vi "Periodic Tasks.vi"(8 "error in":errorcluster) -> ()   [LabVIEW 2017]
doc: "This VI runs in parallel to other tasks. It can contain as many user-defined periodic loops as you need. These can carry out PID or other sorts of timed response."
uses:
  <vilib>/Rock Robotics/WPI/Solenoid/WPI_SolenoidValue.ctl
  <vilib>/Rock Robotics/WPI/ThirdParty/Phoenix-LabVIEW/Motor Controller/Controls/CTRE_Phoenix_MotorControl_ControlMode.ctl
  <vilib>/Rock Robotics/WPI/ThirdParty/Phoenix-LabVIEW/Pigeon IMU/CTRE_PigeonIMU_TareType.ctl
  <vilib>/Rock Robotics/WPI/Utilities/WPI_GetSetVariantRefNum.vi
  Robot Global Data.vi
  <vilib>/Rock Robotics/Network Tables/NT Read Number.vi
  <vilib>/Rock Robotics/Network Tables/NT Write Number.vi
  <vilib>/Rock Robotics/WPI/ThirdParty/Phoenix-LabVIEW/Pigeon IMU/CTRE_PigeonIMU_GetYPR.vi
  <vilib>/Rock Robotics/WPI/ThirdParty/Phoenix-LabVIEW/Motor Controller/Get/CTRE_Phoenix_MotorController_GetSelectedSensorData.vi
  <vilib>/Rock Robotics/WPI/ThirdParty/Phoenix-LabVIEW/Motor Controller/Get/CTRE_Phoenix_MotorController_GetLimitSwitchStates.vi
  <vilib>/Rock Robotics/WPI/Solenoid/WPI_SolenoidSetEnum.vi
  <vilib>/Utility/file.llb/Read Delimited Spreadsheet (DBL).vi
panel:
  out "all rows":dbl[][](array[numeric])
  out "Waveform Chart":dbl(graph)
  in  "HFB_Duration":dbl=200.0
  out "HFB_Start":dbl
  in  "Throttle Correction":bool=TRUE
  in  "Aim-Assist Gain":dbl=0.6
  out "4":dbl(graph)
  out "Current":dbl(graph)
  out "in":i32
  out "ARM":dbl
  out "FWD":bool
  out "Right spd":dbl
  out "Left spd":dbl
  out "Right pos":i32
  out "Left pos":i32
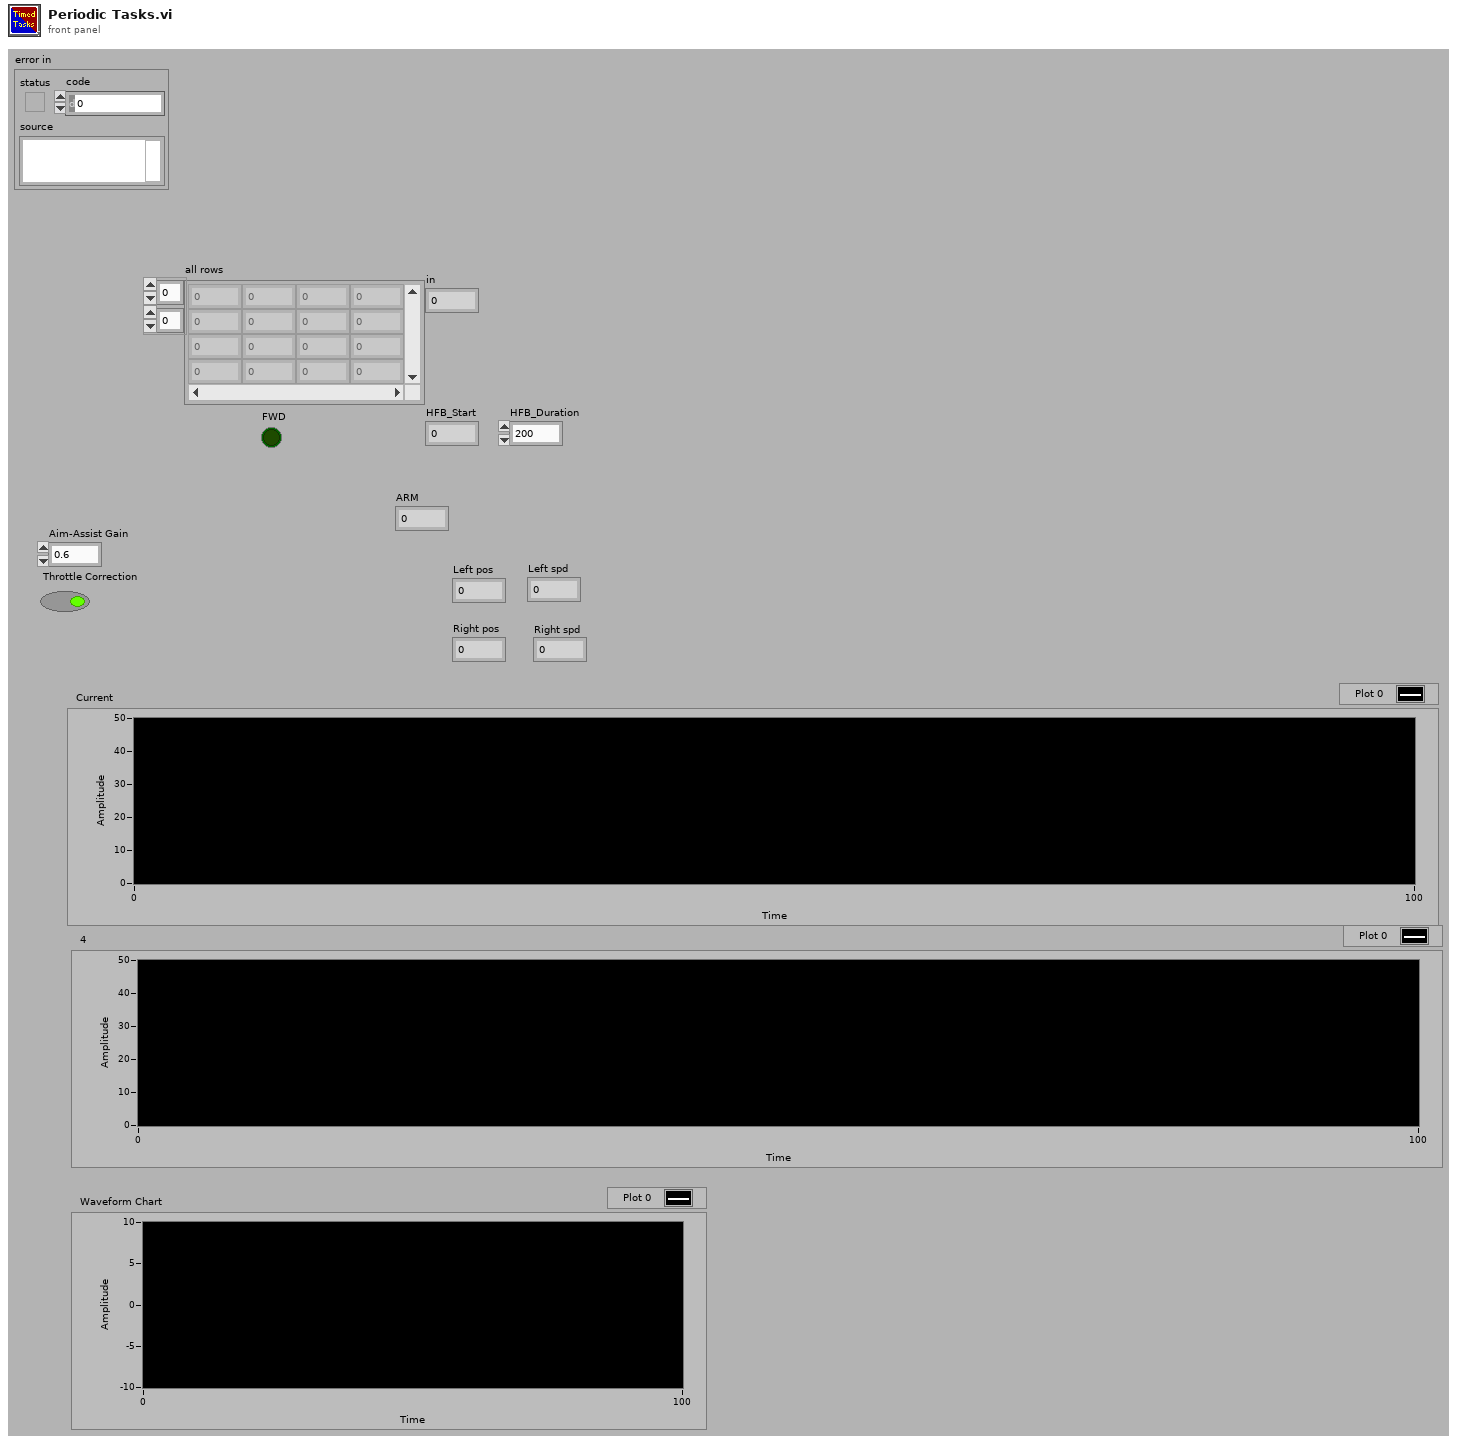
[diagram p1: front panel]
types:
  T1 = typedef "WPI_JoystickDevRef.ctl" = cluster{"Device":T2}
  T2 = typedef "WPI_JoystickDeviceEnum.ctl" = enum16{"USB 0", "USB 1", "USB 2", "USB 3", "USB 4", "USB 5"}
  T3 = typedef "WPI_RobotDriveDevRef.ctl" = cluster{"DevStatus":errorcluster, "Motors[]":T4[], "Square Inputs":bool, "Max Output":dbl}
  T4 = typedef "WPI_MotorControlDeviceRef.ctl" = cluster{"DeviceStatus":errorcluster, "Type":T5, "PWM":cluster{"PWM Channel":T6, "DeadBand":T7}, "CAN":cluster{"Device Number":u8, "SetOutput VI Ref":variant, "GetOutput VI Ref":variant, "Enable VI Ref":variant, "Disable VI Ref":variant, "Data":variant}, "Invert":bool, "DIO PWM":cluster{"PWM \"Enable\" Channel":T6, "DIOChannel":T8, "PWM Rate":dbl}}
  T5 = typedef "WPI_MotorControlType.ctl" = enum16{"PWM", "CAN", "DIO PWM"}
  T6 = typedef "FPGA_DIOPWMChannel.ctl" = enum8{"PWM 0", "PWM 1", "PWM 2", "PWM 3", "PWM 4", "PWM 5", "PWM 6", "PWM 7", "PWM 8", "PWM 9", "PWM MXP 0", "PWM MXP 1", "PWM MXP 2", "PWM MXP 3", "PWM MXP 4", "PWM MXP 5", "PWM MXP 6", "PWM MXP 7", "PWM MXP 8", "PWM MXP 9", "Invalid"}
  T7 = typedef "WPI_PWMDeadband.ctl" = cluster{"Name":string, "maxPositivePwm":i32, "minPositivePwm":i32, "centerPwm":i32, "maxNegativePwm":i32, "minNegativePwm":i32, "angularRange":u16}
  T8 = typedef "FPGA_DIOChannel.ctl" = enum8{"DIO 0", "DIO 1", "DIO 2", "DIO 3", "DIO 4", "DIO 5", "DIO 6", "DIO 7", "DIO 8", "DIO 9", "DIO MXP 0", "DIO MXP 1", "DIO MXP 2", "DIO MXP 3", "DIO MXP 4", "DIO MXP 5", "DIO MXP 6", "DIO MXP 7", "DIO MXP 8", "DIO MXP 9", "DIO MXP 10", "DIO MXP 11", "DIO MXP 12", "DIO MXP 13", "DIO MXP 14", "DIO MXP 15", "SPI Port CS1", "SPI Port CS2", "SPI Port CS3", "SPI Port MISO", "SPI Port MOSI", "Invalid"}
  T9 = typedef "WPI_SolenoidDevRef.ctl" = cluster{"DevStatus":errorcluster, "Pneumatics Control Module":u8, "Forward Solenoid Channel":T10, "Reverse Solenoid Channel":T10}
  T10 = typedef "WPI_SolenoidChannel.ctl" = enum8{"Solenoid 0", "Solenoid 1", "Solenoid 2", "Solenoid 3", "Solenoid 4", "Solenoid 5", "Solenoid 6", "Solenoid 7", "Invalid"}
  T11 = typedef "CTRE_PigeonIMU_DeviceRef.ctl" = cluster{"DeviceStatus":errorcluster, "Device Number":u8, "Type":T12, "Device ID":u32, "Handle":u64, "UsageFrame":u32, "Library Path":path}
  T12 = typedef "CTRE_PigeonIMU_ConnectionType.ctl" = u32
  T13 = cluster{"JoystickDevRef":T1, "JoystickDevRef":T1, "RobotDriveDevRef":T3, "PhoenixMotorControlDevRef":T4, "SolenoidDevRef":T9, "PhoenixMotorControlDevRef":T4, "SolenoidDevRef":T9, "SolenoidDevRef":T9, "PhoenixMotorControlDevRef":T4, "PhoenixMotorControlDevRef":T4, "SolenoidDevRef":T9, "PhoenixMotorControlDevRef":T4, "PhoenixMotorControlDevRef":T4, "PigeonIMUDevRef":T11, "SolenoidDevRef":T9, "Name":string, "Name":string, "Name":string, "Name":string}
  T14 = typedef "CTRE_PigeonIMU_TareType.ctl" = u8
  T15 = typedef "WPI_DriverStationRobotMode2.ctl" = enum16{"Autonomous Disabled", "Autonomous Enabled", "Teleop Disabled", "Teleop Enabled", "Disconnected", "Finish", "Test Disabled", "Test Enabled", "Emergency Stopped"}
  T16 = typedef "WPI_SolenoidValue.ctl" = enum16{"Off", "On", "Forward", "Reverse"}
  T17 = typedef "CTRE_Phoenix_MotorControl_ControlMode.ctl" = u16
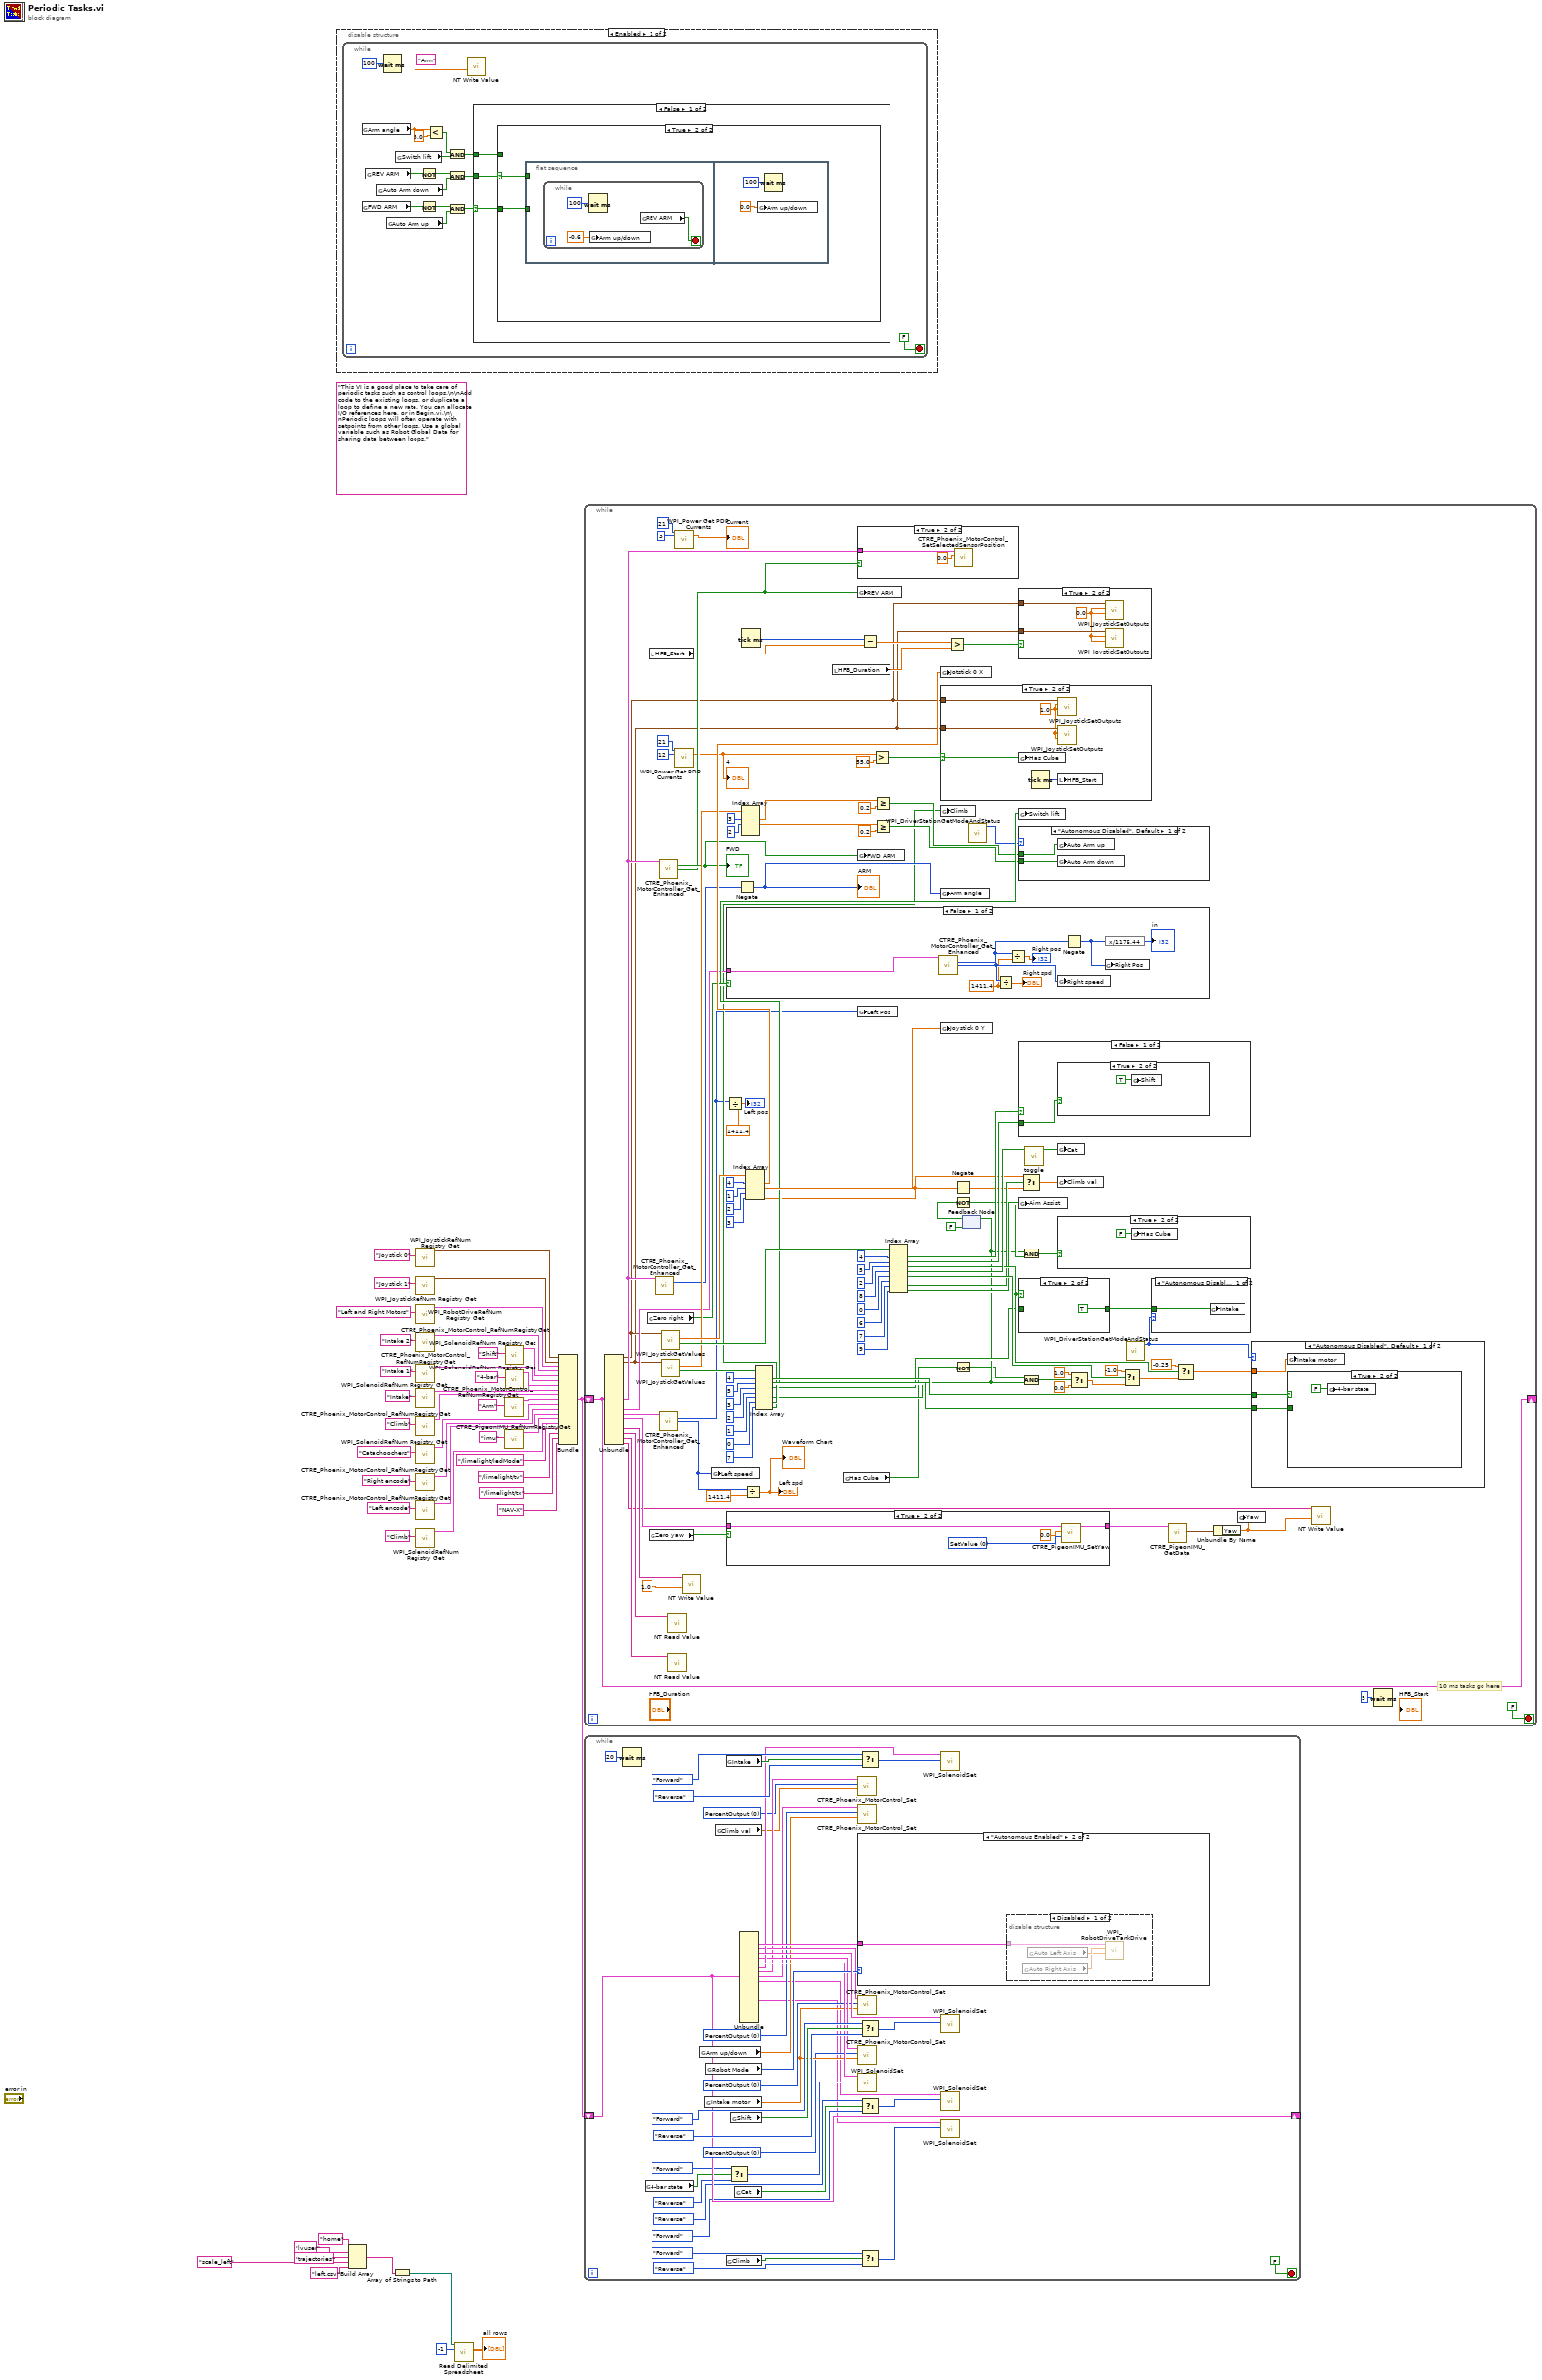
[diagram p0: block diagram]
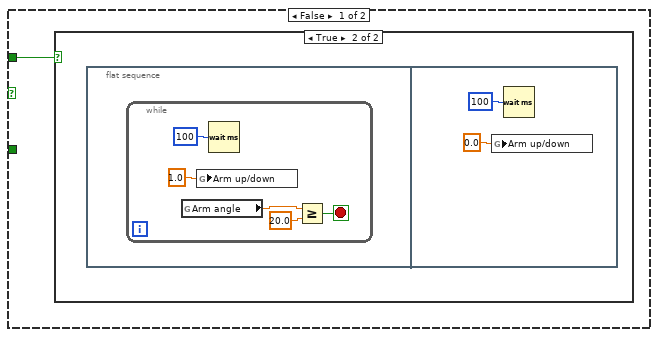
[diagram p2: hidden frame]
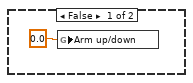
[diagram p3: hidden frame]
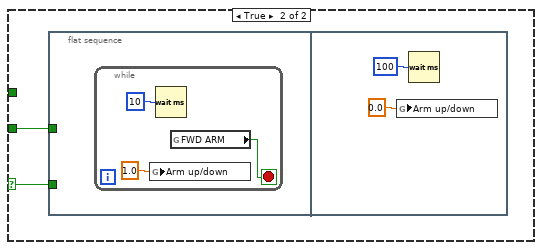
[diagram p4: hidden frame]
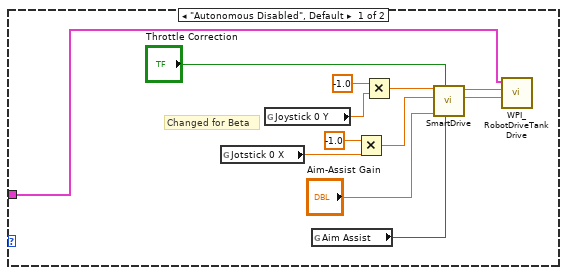
[diagram p6: hidden frame]
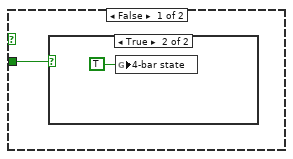
[diagram p14: hidden frame]
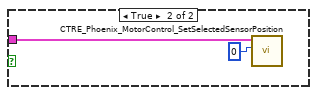
[diagram p19: hidden frame]
diagram:
  (unwired) "This VI is a good place to take care of periodic tasks such as control loops.\n\nAdd code to the existing loops, or duplicate a loop to define a new rate. You can allocate I/O references here, or in Begin.vi.\n\nPeriodic loops will often operate with setpoints from other loops. Use a global variable such as Robot Global Data for sharing data between loops."
  n1 = disable-structure shown="Enabled" {
    frame Enabled {
      n2 = while {
        stop <- FALSE stop-if-true
        n3 = global read "Robot Global Data.vi" "Arm angle"() -> (w54:dbl)
        n4 = global read "Robot Global Data.vi" "FWD ARM"() -> (w46:bool)
        n5 = global read "Robot Global Data.vi" "REV ARM"() -> (w48:bool)
        n6 = global read "Robot Global Data.vi" "Auto Arm down"() -> (w50:bool)
        n7 = Wait (ms)(milliseconds to wait=u32 100) -> ()  [unwired: 1 out]
        n8 = global read "Robot Global Data.vi" "Auto Arm up"() -> (w52:bool)
        n9 = global read "Robot Global Data.vi" "Switch lift"() -> (w56:bool)
        n10 = Not(x=w48) -> (.not. x?=w47:bool)
        n11 = Not(x=w46) -> (.not. x?=w45:bool)
        n12 = Less?(x=w54, y=5.0) -> (x < y?=w57:bool)
        n13 = And(x=w57, y=w56) -> (x .and. y?=w55:bool)
        n14 = Compound Arithmetic op=AND(w47, w50) -> (w49:bool)
        n15 = Compound Arithmetic op=AND(w45, w52) -> (w51:bool)
        n16 = call-poly <vilib>:"NT Write Value.vi"("Numeric"=w54, "Name"="Arm") -> ()  [unwired: 9 in, 1 out]
        n17 = case shown="False" w51 {
          selector: w51 -> [w62 w80]
          tunnel: w49 -> [w63 w81]
          tunnel: w55 -> [w61 _]
          frame False {
            n18 = case shown="True" w63 {
              selector: w63 -> [_ w74]
              tunnel: w62 -> [_ w73]
              tunnel: w61 -> [w64 _]
              frame False {
                n19 = case shown="True" w64 {
                  frame False {
                    n20 = global write "Robot Global Data.vi" "Arm up/down"(0.0 ("Arm up/down")) -> ()
                  }
                  frame True {
                    n21 = flat-sequence {
                      frame #0 {
                        n22 = while {
                          stop <- w67 stop-if-true
                          n23 = global read "Robot Global Data.vi" "Arm angle"() -> (w69:dbl)
                          n24 = global write "Robot Global Data.vi" "Arm up/down"(1.0) -> ()
                          n25 = Wait (ms)(milliseconds to wait=u32 100) -> ()  [unwired: 1 out]
                          n26 = Greater Or Equal?(x=w69, y=20.0) -> (x >= y?=w67:bool)
                        }
                      }
                      frame #1 {
                        n27 = global write "Robot Global Data.vi" "Arm up/down"(0.0) -> ()
                        n28 = Wait (ms)(milliseconds to wait=u32 100) -> ()  [unwired: 1 out]
                      }
                    }
                  }
                }
              }
              frame True {
                n29 = flat-sequence {
                  tunnel: w74 -> [_]
                  tunnel: w73 -> [_]
                  frame #0 {
                    n30 = while {
                      stop <- w75 stop-if-true
                      n31 = Wait (ms)(milliseconds to wait=u32 100) -> ()  [unwired: 1 out]
                      n32 = global write "Robot Global Data.vi" "Arm up/down"(-0.6) -> ()
                      n33 = global read "Robot Global Data.vi" "REV ARM"() -> (w75:bool)
                    }
                  }
                  frame #1 {
                    n34 = global write "Robot Global Data.vi" "Arm up/down"(0.0) -> ()
                    n35 = Wait (ms)(milliseconds to wait=u32 100) -> ()  [unwired: 1 out]
                  }
                }
              }
            }
          }
          frame True {
            n36 = flat-sequence {
              tunnel: w81 -> [_]
              tunnel: w80 -> [_]
              frame #0 {
                n37 = while {
                  stop <- w82 stop-if-true
                  n38 = global write "Robot Global Data.vi" "Arm up/down"(1.0) -> ()
                  n39 = Wait (ms)(milliseconds to wait=u32 10) -> ()  [unwired: 1 out]
                  n40 = global read "Robot Global Data.vi" "FWD ARM"() -> (w82:bool)
                }
              }
              frame #1 {
                n41 = global write "Robot Global Data.vi" "Arm up/down"(0.0) -> ()
                n42 = Wait (ms)(milliseconds to wait=u32 100) -> ()  [unwired: 1 out]
              }
            }
          }
        }
      }
    }
    frame Disabled {
    }
  }
  n43 = Build Array("home", "lvuser" ("element"), "trajectories" ("element"), "scale_left" ("element"), "left.csv" ("element")) -> (w3:string[])
  n44 = Array of Strings to Path(0:w3) -> (2:w2:path)  [unwired: 1 in]
  n45 = call <vilib>:"WPI_JoystickRefNum Registry Get.vi"("refnum name"="Joystick 0") -> ("JoystickDevRef"=w32:T1)  [unwired: 1 in, 9 out]
  n46 = call <vilib>:"WPI_JoystickRefNum Registry Get.vi"("refnum name"="Joystick 1") -> ("JoystickDevRef"=w42:T1)  [unwired: 1 in, 9 out]
  n47 = call <vilib>:"WPI_RobotDriveRefNum Registry Get.vi"("refnum name"="Left and Right Motors") -> ("RobotDriveDevRef"=w41:T3)  [unwired: 1 in, 9 out]
  n48 = call <vilib>:"CTRE_Phoenix_MotorControl_RefNumRegistryGet.vi"("refnum name"="Intake 2") -> ("PhoenixMotorControlDevRef"=w38:T4)  [unwired: 9 in, 1 out]
  n49 = call <vilib>:"CTRE_Phoenix_MotorControl_RefNumRegistryGet.vi"("refnum name"="Intake 1") -> ("PhoenixMotorControlDevRef"=w35:T4)  [unwired: 9 in, 1 out]
  n50 = call <vilib>:"WPI_SolenoidRefNum Registry Get.vi"("refnum name"="Intake") -> ("SolenoidDevRef"=w30:T9)  [unwired: 9 in, 1 out]
  n51 = call <vilib>:"CTRE_Phoenix_MotorControl_RefNumRegistryGet.vi"("refnum name"="Climb") -> ("PhoenixMotorControlDevRef"=w26:T4)  [unwired: 9 in, 1 out]
  n52 = call <vilib>:"WPI_SolenoidRefNum Registry Get.vi"("refnum name"="Catachoochers") -> ("SolenoidDevRef"=w22:T9)  [unwired: 9 in, 1 out]
  n53 = call <vilib>:"CTRE_Phoenix_MotorControl_RefNumRegistryGet.vi"("refnum name"="Right encode") -> ("PhoenixMotorControlDevRef"=w20:T4)  [unwired: 9 in, 1 out]
  n54 = call <vilib>:"CTRE_Phoenix_MotorControl_RefNumRegistryGet.vi"("refnum name"="Left encode") -> ("PhoenixMotorControlDevRef"=w18:T4)  [unwired: 9 in, 1 out]
  n55 = call <vilib>:"WPI_SolenoidRefNum Registry Get.vi"("refnum name"="Climb") -> ("SolenoidDevRef"=w14:T9)  [unwired: 9 in, 1 out]
  n56 = call-poly <vilib>:"Read Delimited Spreadsheet.vi"("file path (dialog if empty)"=w2, "number of rows (all:-1)"=-1) -> ("all rows"=→"all rows":dbl[][])  [unwired: 8 in, 5 out]
  n57 = call <vilib>:"CTRE_Phoenix_MotorControl_RefNumRegistryGet.vi"("refnum name"="Arm") -> ("PhoenixMotorControlDevRef"=w24:T4)  [unwired: 9 in, 1 out]
  n58 = call <vilib>:"CTRE_PigeonIMU_RefNumRegistryGet.vi"("refnum name"="imu") -> ("PigeonIMUDevRef"=w17:T11)  [unwired: 9 in, 1 out]
  n59 = call <vilib>:"WPI_SolenoidRefNum Registry Get.vi"("refnum name"="Shift") -> ("SolenoidDevRef"=w36:T9)  [unwired: 9 in, 1 out]
  n60 = call <vilib>:"WPI_SolenoidRefNum Registry Get.vi"("refnum name"="4-bar") -> ("SolenoidDevRef"=w31:T9)  [unwired: 9 in, 1 out]
  n61 = Bundle("JoystickDevRef"=w32, "JoystickDevRef"=w42, "RobotDriveDevRef"=w41, "PhoenixMotorControlDevRef"=w38, "SolenoidDevRef"=w36, "PhoenixMotorControlDevRef"=w35, "SolenoidDevRef"=w31, "SolenoidDevRef"=w30, "PhoenixMotorControlDevRef"=w26, "PhoenixMotorControlDevRef"=w24, "SolenoidDevRef"=w22, "PhoenixMotorControlDevRef"=w20, "PhoenixMotorControlDevRef"=w18, "PigeonIMUDevRef"=w17, "SolenoidDevRef"=w14, "Name"="/limelight/ledMode", "Name"="/limelight/tv", "Name"="/limelight/tx", "Name"="NAV-X") -> (w40:T13)  [unwired: 1 out]
  n62 = while {
    shift-right: [w186] -> _
    shift-left: w40 -> [w186]
    stop <- FALSE stop-if-true
    # "10 ms tasks go here"
    n63 = Unbundle(w186) -> ("JoystickDevRef"=w98:T1, "JoystickDevRef"=w97:T1, "PhoenixMotorControlDevRef"=w138:T4, "PhoenixMotorControlDevRef"=w143:T4, "PhoenixMotorControlDevRef"=w142:T4, "PigeonIMUDevRef"=w133:T11, "Name"=w96:string, "Name"=w95:string, "Name"=w94:string, "Name"=w93:string)  [unwired: 9 out]
    n64 = global read "Robot Global Data.vi" "Zero right"() -> (w162:bool)
    n65 = local read "HFB_Start"() -> (w102:dbl)
    n66 = global read "Robot Global Data.vi" "Zero yaw"() -> (w131:bool)
    n67 = call-poly <vilib>:"CTRE_Phoenix_MotorController_Get_Enhanced.vi"("PhoenixMotorControlDevRef"=w138) -> ("Position (Raw Sensor Units)"=w137:i32)  [unwired: 11 in, 3 out]
    n68 = call-poly <vilib>:"CTRE_Phoenix_MotorController_Get_Enhanced.vi"("PhoenixMotorControlDevRef"=w138) -> ("Forward Limit Closed?"=w135:bool, "Reverse Limit Closed?"=w134:bool)  [unwired: 11 in, 2 out]
    "FWD" <- w135
    n69 = call-poly <vilib>:"CTRE_Phoenix_MotorController_Get_Enhanced.vi"("PhoenixMotorControlDevRef"=w142) -> ("Position (Raw Sensor Units)"=w88:i32, "Velocity (Raw Sensor Units per 100 ms)"=w92:i32)  [unwired: 11 in, 2 out]
    n70 = call <vilib>:"WPI_JoystickGetValues.vi"("JoystickDevRef"=w98) -> ("Buttons"=w185:bool[], "Axes"=w193:dbl[])  [unwired: 6 in, 3 out]
    n71 = call <vilib>:"WPI_JoystickGetValues.vi"("JoystickDevRef"=w97) -> ("Buttons"=w182:bool[], "Axes"=w167:dbl[])  [unwired: 6 in, 3 out]
    n72 = call-poly <vilib>:"NT Read Value.vi"("Name"=w95) -> ()  [unwired: 9 in, 2 out]
    n73 = call-poly <vilib>:"NT Read Value.vi"("Name"=w94) -> ()  [unwired: 9 in, 2 out]
    n74 = call <vilib>:"WPI_Power Get PDP Currents.vi"("Power Distribution Panel (0)"=u8 21, "PDP Channel"=3) -> ("current (A)"=→"Current":dbl)  [unwired: 11 in, 2 out]
    n75 = call <vilib>:"WPI_Power Get PDP Currents.vi"("Power Distribution Panel (0)"=u8 21, "PDP Channel"=12) -> ("current (A)"=w106:dbl)  [unwired: 11 in, 2 out]
    "4" <- w106
    n76 = call-poly <vilib>:"NT Write Value.vi"("Numeric"=1.0, "Name"=w96) -> ()  [unwired: 9 in, 1 out]
    n77 = global write "Robot Global Data.vi" "Left speed"(w92) -> ()
    n78 = case shown="False" w162 {
      tunnel: w143 -> [w230 w232]
      frame False {
        w223 = 1411.4 ("y")
        n79 = call-poly <vilib>:"CTRE_Phoenix_MotorController_Get_Enhanced.vi"("PhoenixMotorControlDevRef"=w230) -> ("Position (Raw Sensor Units)"=w224:i32, "Velocity (Raw Sensor Units per 100 ms)"=w226:i32)  [unwired: 11 in, 2 out]
        n80 = Divide(x=w226, y=w223) -> (x/y=→"Right spd":dbl)
        n81 = Divide(x=w224, y=w223) -> (x/y=→"Right pos":dbl)
        n82 = global write "Robot Global Data.vi" "Right speed"(w226) -> ()
        n83 = Negate(x=w224) -> (-x=w229:i32)
        n84 = expression code="x/1176.44"(w229) -> (→"in":i32)
        n85 = global write "Robot Global Data.vi" "Right Pos"(w229) -> ()
      }
      frame True {
        n86 = call <vilib>:"CTRE_Phoenix_MotorControl_SetSelectedSensorPosition.vi"("New Sensor Position"=0, "PhoenixMotorControlDevRef"=w232) -> ()  [unwired: 8 in, 2 out]
      }
    }
    n87 = Divide(x=w88, y=1411.4) -> (x/y=→"Left pos":dbl)
    n88 = case shown="True" w131 {
      tunnel: w133 -> [w206 w208]
      tunnel: [w206 w207] -> w132
      frame False {
      }
      frame True {
        w210 = T14 0 items=["SetValue"=0, "AddOffset"=1, "MatchCompass"=2, "SetOffset"=255] ("TareType (SetValue)")
        n89 = call <vilib>:"CTRE_PigeonIMU_SetYaw.vi"("TareType (SetValue)"=w210, "Value"=0.0, "PigeonIMUDevRef"=w208) -> ("PigeonIMUDevRef"=w207:T11)  [unwired: 7 in, 1 out]
      }
    }
    n90 = Negate(x=w137) -> (-x=w136:i32)
    "ARM" <- w136
    n91 = Index Array(array=w167, index #1=3 ("index"), index #2=2 ("index")) -> (element #1=w161:dbl, element #2=w159:dbl)  [unwired: 2 in, 2 out]
    n92 = Tick Count (ms)() -> (millisecond timer value=w103:u32)
    n93 = Divide(x=w92, y=1411.4) -> (x/y=→"Left spd" →"Waveform Chart":dbl)
    n94 = Index Array(array=w193, index #1=4 ("index"), index #2=1 ("index"), index #3=2 ("index"), index #4=3 ("index")) -> (element #1=w190:dbl, element #2=w189:dbl, element #4=w126:dbl)  [unwired: 1 out]
    n95 = Index Array(array=w182, index #1=4 ("index"), index #2=5 ("index"), index #3=3 ("index"), index #4=2 ("index"), index #5=1 ("index"), index #6=0 ("index"), index #7=7 ("index")) -> (element #1=w179:bool, element #2=w178:bool, element #3=w145:bool, element #5=w109:bool, element #6=w152:bool, element #7=w129:bool)  [unwired: 1 out]
    n96 = local read "HFB_Duration"() -> (w100:dbl)
    n97 = global read "Robot Global Data.vi" "Has Cube"() -> (w108:bool)
    n98 = case shown="True" w134 {
      tunnel: w138 -> [_ w212]
      frame False {
      }
      frame True {
        n99 = call <vilib>:"CTRE_Phoenix_MotorControl_SetSelectedSensorPosition.vi"("New Sensor Position"=0.0 ("Output"), "PhoenixMotorControlDevRef"=w212) -> ()  [unwired: 8 in, 2 out]
      }
    }
    n100 = global write "Robot Global Data.vi" "REV ARM"(w134) -> ()
    n101 = global write "Robot Global Data.vi" "FWD ARM"(w135) -> ()
    n102 = global write "Robot Global Data.vi" "Left Pos"(w88) -> ()
    n103 = Subtract(x=w103, y=w102) -> (x-y=w101:dbl)
    n104 = Greater?(x=w106, y=55.0) -> (0:w104:bool)
    n105 = Greater Or Equal?(x=w161, y=0.2) -> (x >= y?=w148:bool)
    n106 = Greater Or Equal?(x=w159, y=0.2) -> (x >= y?=w147:bool)
    n107 = Index Array(array=w185, index #1=4 ("index"), index #2=5 ("index"), index #3=2 ("index"), index #4=8 ("index"), index #5=0 ("index"), index #6=6 ("index"), index #7=7 ("index"), index #8=9) -> (element #1=w184:bool, element #2=w183:bool, element #3=w146:bool, element #4=w163:bool, element #5=w156:bool, element #7=w127:bool, element #8=w116:bool)  [unwired: 1 out]
    n108 = global write "Robot Global Data.vi" "Jotstick 0 X"(w190) -> ()
    n109 = case shown="True" w104 {
      selector: w104 -> [_ w203]
      tunnel: w98 -> [_ w201]
      tunnel: w97 -> [_ w200]
      frame False {
      }
      frame True {
        w199 = sgl 1.0 ("Left Rumble")
        n110 = global write "Robot Global Data.vi" "Has Cube"(w203) -> ()
        n111 = Tick Count (ms)() -> (millisecond timer value=w202:u32)
        n112 = call <vilib>:"WPI_JoystickSetOutputs.vi"("Right Rumble"=w199, "Left Rumble"=w199, "JoystickDevRef"=w201) -> ()  [unwired: 7 in, 2 out]
        n113 = call <vilib>:"WPI_JoystickSetOutputs.vi"("Right Rumble"=w199, "Left Rumble"=w199, "JoystickDevRef"=w200) -> ()  [unwired: 7 in, 2 out]
        n114 = local write "HFB_Start"(w202) -> ()
      }
    }
    n115 = global write "Robot Global Data.vi" "Climb"(w129) -> ()
    n116 = global write "Robot Global Data.vi" "Arm angle"(w136) -> ()
    n117 = global write "Robot Global Data.vi" "Joystick 0 Y"(w189) -> ()
    n118 = Greater?(x=w101, y=w100) -> (0:w99:bool)
    n119 = Negate(x=w126) -> (-x=w125:dbl)
    n120 = Not(x=w108) -> (.not. x?=w107:bool)
    n121 = feedback-in #1(w109) -> ()
    n122 = feedback #1(FALSE) -> (w114:bool)
    n123 = Not(x=w114) -> (.not. x?=w113:bool)
    n124 = call <vilib>:"WPI_DriverStationGetModeAndStatus.vi"() -> ("Robot Mode"=w149:T15)  [unwired: 10 in, 1 out]
    n125 = case shown="True" w99 {
      tunnel: w98 -> [_ w198]
      tunnel: w97 -> [_ w197]
      frame False {
      }
      frame True {
        w196 = sgl 0.0 ("Left Rumble")
        n126 = call <vilib>:"WPI_JoystickSetOutputs.vi"("Right Rumble"=w196, "Left Rumble"=w196, "JoystickDevRef"=w198) -> ()  [unwired: 7 in, 2 out]
        n127 = call <vilib>:"WPI_JoystickSetOutputs.vi"("Right Rumble"=w196, "Left Rumble"=w196, "JoystickDevRef"=w197) -> ()  [unwired: 7 in, 2 out]
      }
    }
    n128 = global write "Robot Global Data.vi" "Switch lift"(w152) -> ()
    n129 = case shown="\"Autonomous Disabled\", Default" w149 {
      tunnel: w148 -> [w222 _]
      tunnel: w147 -> [w221 _]
      frame "Autonomous Disabled", Default {
        n130 = global write "Robot Global Data.vi" "Auto Arm up"(w222) -> ()
        n131 = global write "Robot Global Data.vi" "Auto Arm down"(w221) -> ()
      }
      frame "Autonomous Enabled" {
      }
    }
    n132 = case shown="False" w184 {
      tunnel: w183 -> [w233 _]
      frame False {
        n133 = case shown="True" w233 {
          frame False {
          }
          frame True {
            n134 = global write "Robot Global Data.vi" "Shift"(TRUE) -> ()
          }
        }
      }
      frame True {
        n135 = global write "Robot Global Data.vi" "Shift"(FALSE) -> ()
      }
    }
    n136 = global write "Robot Global Data.vi" "Aim Assist"(w116) -> ()
    n137 = case shown="True" w146 {
      tunnel: w145 -> [w219 _]
      tunnel: [w219 TRUE] -> w144
      frame False {
      }
      frame True {
      }
    }
    n138 = Select(t=w126, s=w127, f=w125) -> (s? t:f=w124:dbl)
    n139 = And(x=w109, y=w113) -> (x .and. y?=w111:bool)
    n140 = And(x=w107, y=w109) -> (x .and. y?=w110:bool)
    n141 = call "toggle.vi"("Boolean"=w163) -> ("Boolean 2"=w154:bool)  [unwired: 10 in]
    n142 = global write "Robot Global Data.vi" "Cat"(w154) -> ()
    n143 = global write "Robot Global Data.vi" "Climb val"(w124) -> ()
    n144 = case shown="True" w111 {
      frame False {
      }
      frame True {
        n145 = global write "Robot Global Data.vi" "Has Cube"(FALSE) -> ()
      }
    }
    n146 = Select(t=1.0, s=w110, f=0.0) -> (s? t:f=w173:dbl)
    n147 = Select(t=-1.0, s=w156, f=w173) -> (s? t:f=w150:dbl)
    n148 = call <vilib>:"WPI_DriverStationGetModeAndStatus.vi"() -> ("Robot Mode"=w115:T15)  [unwired: 10 in, 1 out]
    n149 = case shown="\"Autonomous Disabled\", Default" w115 {
      tunnel: w144 -> [w205 _]
      frame "Autonomous Disabled", Default {
        n150 = global write "Robot Global Data.vi" "Intake"(w205) -> ()
      }
      frame "Autonomous Enabled" {
      }
    }
    n151 = call-poly <vilib>:"CTRE_PigeonIMU_GetData.vi"("PigeonIMUDevRef"=w132) -> ("Yaw Pitch Roll"=w141:cluster{"Yaw":dbl, "Pitch":dbl, "Roll":dbl})  [unwired: 8 in, 2 out]
    n152 = Select(t=-0.25, s=w146, f=w150) -> (s? t:f=w123:dbl)
    n153 = Unbundle By Name(w141) -> ("Yaw"=w140:dbl)
    n154 = global write "Robot Global Data.vi" "Yaw"(w140) -> ()
    n155 = case shown="\"Autonomous Disabled\", Default" w115 {
      tunnel: w179 -> [w215 _]
      tunnel: w178 -> [w214 _]
      tunnel: w123 -> [w213 _]
      frame "Autonomous Disabled", Default {
        n156 = global write "Robot Global Data.vi" "Intake motor"(w213) -> ()
        n157 = case shown="True" w215 {
          tunnel: w214 -> [w216 _]
          frame False {
            n158 = case shown="True" w216 {
              frame False {
              }
              frame True {
                n159 = global write "Robot Global Data.vi" "4-bar state"(TRUE) -> ()
              }
            }
          }
          frame True {
            n160 = global write "Robot Global Data.vi" "4-bar state"(FALSE) -> ()
          }
        }
      }
      frame "Autonomous Enabled" {
      }
    }
    n161 = call-poly <vilib>:"NT Write Value.vi"("Numeric"=w140, "Name"=w93) -> ()  [unwired: 9 in, 1 out]
    n162 = Wait (ms)(milliseconds to wait=u32 5) -> ()  [unwired: 1 out]
  }
  n163 = while {
    shift-right: [w270] -> _
    shift-left: w40 -> [w270]
    stop <- FALSE stop-if-true
    w248 = T17 0 items=["PercentOutput"=0, "Position"=1, "Velocity"=2, "Current"=3, "Follower"=5, "MotionProfile"=6, "MotionMagic"=7, "MotionMagicArc"=8, "MotionProfileArc"=10, "Disabled"=15] ("Control Mode")
    w250 = T17 0 items=["PercentOutput"=0, "Position"=1, "Velocity"=2, "Current"=3, "Follower"=5, "MotionProfile"=6, "MotionMagic"=7, "MotionMagicArc"=8, "MotionProfileArc"=10, "Disabled"=15] ("Control Mode")
    w252 = T17 0 items=["PercentOutput"=0, "Position"=1, "Velocity"=2, "Current"=3, "Follower"=5, "MotionProfile"=6, "MotionMagic"=7, "MotionMagicArc"=8, "MotionProfileArc"=10, "Disabled"=15] ("Control Mode")
    w253 = T17 0 items=["PercentOutput"=0, "Position"=1, "Velocity"=2, "Current"=3, "Follower"=5, "MotionProfile"=6, "MotionMagic"=7, "MotionMagicArc"=8, "MotionProfileArc"=10, "Disabled"=15] ("Control Mode")
    n164 = Wait (ms)(milliseconds to wait=u32 20) -> ()  [unwired: 1 out]
    n165 = global read "Robot Global Data.vi" "4-bar state"() -> (w266:bool)
    n166 = global read "Robot Global Data.vi" "Arm up/down"() -> (w247:dbl)
    n167 = global read "Robot Global Data.vi" "Intake motor"() -> (w254:dbl)
    n168 = global read "Robot Global Data.vi" "Robot Mode"() -> (w268:T15)
    n169 = global read "Robot Global Data.vi" "Climb val"() -> (w236:dbl)
    n170 = global read "Robot Global Data.vi" "Intake"() -> (w261:bool)
    n171 = global read "Robot Global Data.vi" "Climb"() -> (w237:bool)
    n172 = Select(t=WPI_SolenoidValue."Forward" ("Value"), s=w266, f=WPI_SolenoidValue."Reverse" ("Value")) -> (s? t:f=w263:T16)
    n173 = global read "Robot Global Data.vi" "Shift"() -> (w272:bool)
    n174 = global read "Robot Global Data.vi" "Cat"() -> (w242:bool)
    n175 = Unbundle(w270) -> ("RobotDriveDevRef"=w267:T3, "PhoenixMotorControlDevRef"=w256:T4, "SolenoidDevRef"=w269:T9, "PhoenixMotorControlDevRef"=w255:T4, "SolenoidDevRef"=w262:T9, "SolenoidDevRef"=w257:T9, "PhoenixMotorControlDevRef"=w251:T4, "PhoenixMotorControlDevRef"=w249:T4, "SolenoidDevRef"=w243:T9, "SolenoidDevRef"=w241:T9)  [unwired: 9 out]
    n176 = call <vilib>:"CTRE_Phoenix_MotorControl_Set.vi"("Output"=w236, "Control Mode"=w250, "PhoenixMotorControlDevRef"=w251) -> ()  [unwired: 7 in, 2 out]
    n177 = call <vilib>:"CTRE_Phoenix_MotorControl_Set.vi"("Output"=w247, "Control Mode"=w248, "PhoenixMotorControlDevRef"=w249) -> ()  [unwired: 7 in, 2 out]
    n178 = case shown="\"Autonomous Enabled\"" w268 {
      tunnel: w267 -> [w287 w289]
      frame "Autonomous Disabled", Default {
        # "Changed for Beta"
        n179 = global read "Robot Global Data.vi" "Jotstick 0 X"() -> (w282:dbl)
        n180 = global read "Robot Global Data.vi" "Joystick 0 Y"() -> (w277:dbl)
        n181 = global read "Robot Global Data.vi" "Aim Assist"() -> (w284:bool)
        n182 = Multiply(x=-1.0, y=w282) -> (x*y=w280:dbl)
        n183 = Multiply(x=-1.0, y=w277) -> (x*y=w278:dbl)
        n184 = call "SmartDrive.vi"("Aim-Assist"=w284, "Throttle Correction"="Throttle Correction", "Aim-Assist Gain"="Aim-Assist Gain", "Turn"=w280, "Power"=w278) -> ("Magnitude Right"=w285:dbl, "Magnitude Left"=w286:dbl)  [unwired: 5 in]
        n185 = call <vilib>:"WPI_RobotDriveTankDrive.vi"("Right axis value"=w285, "Left axis value"=w286, "RobotDriveDevRef"=w287) -> ()  [unwired: 6 in, 3 out]
      }
      frame "Autonomous Enabled" {
        n186 = disable-structure shown="Disabled" {
          disable-tunnel: w289 -> [w292 _]
          frame Disabled {
            n187 = global read "Robot Global Data.vi" "Auto Right Axis"() -> (w290:dbl)
            n188 = global read "Robot Global Data.vi" "Auto Left Axis"() -> (w291:dbl)
            n189 = call <vilib>:"WPI_RobotDriveTankDrive.vi"("Right axis value"=w290, "Left axis value"=w291, "RobotDriveDevRef"=w292) -> ()  [unwired: 6 in, 3 out]
          }
          frame Enabled {
          }
        }
      }
    }
    n190 = call <vilib>:"CTRE_Phoenix_MotorControl_Set.vi"("Output"=w254, "Control Mode"=w252, "PhoenixMotorControlDevRef"=w256) -> ()  [unwired: 7 in, 2 out]
    n191 = call <vilib>:"CTRE_Phoenix_MotorControl_Set.vi"("Output"=w254, "Control Mode"=w253, "PhoenixMotorControlDevRef"=w255) -> ()  [unwired: 7 in, 2 out]
    n192 = call-poly <vilib>:"WPI_SolenoidSet.vi"("Value"=w263, "SolenoidDevRef"=w262) -> ()  [unwired: 8 in, 2 out]
    n193 = Select(t=WPI_SolenoidValue."Forward" ("Value"), s=w261, f=WPI_SolenoidValue."Reverse" ("Value")) -> (s? t:f=w258:T16)
    n194 = Select(t=WPI_SolenoidValue."Forward" ("Value"), s=w272, f=WPI_SolenoidValue."Reverse" ("Value")) -> (s? t:f=w271:T16)
    n195 = Select(t=WPI_SolenoidValue."Reverse" ("Value"), s=w242, f=WPI_SolenoidValue."Forward" ("Value")) -> (s? t:f=w244:T16)
    n196 = Select(t=WPI_SolenoidValue."Forward" ("Value"), s=w237, f=WPI_SolenoidValue."Reverse" ("Value")) -> (s? t:f=w238:T16)
    n197 = call-poly <vilib>:"WPI_SolenoidSet.vi"("Value"=w258, "SolenoidDevRef"=w257) -> ()  [unwired: 8 in, 2 out]
    n198 = call-poly <vilib>:"WPI_SolenoidSet.vi"("Value"=w271, "SolenoidDevRef"=w269) -> ()  [unwired: 8 in, 2 out]
    n199 = call-poly <vilib>:"WPI_SolenoidSet.vi"("Value"=w244, "SolenoidDevRef"=w243) -> ()  [unwired: 8 in, 2 out]
    n200 = call-poly <vilib>:"WPI_SolenoidSet.vi"("Value"=w238, "SolenoidDevRef"=w241) -> ()  [unwired: 8 in, 2 out]
  }
